vi "Get_reference_samplingdata.vi"(0 "SPU":refnum<k24>, 1 "Ref_monitordata_struct":refnum<k24>[](array[refnum]), 2 "TSL":refnum<k24>, 3 "MPM":refnum<k24>[](array[refnum]), 4 "SOP":i32, 5 "错误输入（无错误）":errorcluster, 6 "STSProcess.PDLSTS":refnum<k24>, 10 "Refdata_struct":refnum<k24>[](array[refnum])) -> (15 "PDLSTS out":refnum<k24>, 19 "error out":errorcluster)   [LabVIEW 2017]
doc: "Get logging reference data & add in"
uses:
  D:/test/PDLSTS/LV_PDL LvVer17.0/LV_PDL_x86/DLL/STSProcess.dll
  DLL/STSProcess.dll
  D:/test/PDLSTS/LV_PDL LvVer17.0/LV_PDL_x86/DLL/InstrumentDLL.dll
  DLL/InstrumentDLL.dll
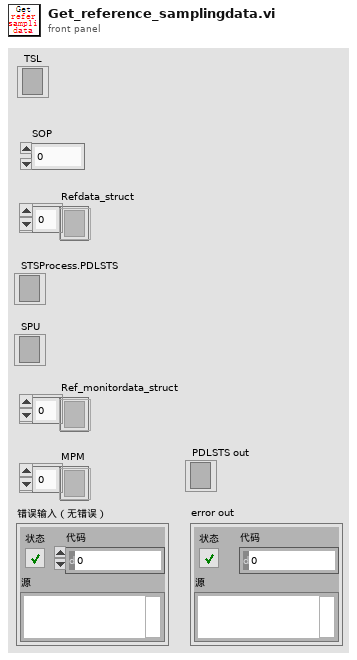
[diagram p1: front panel]
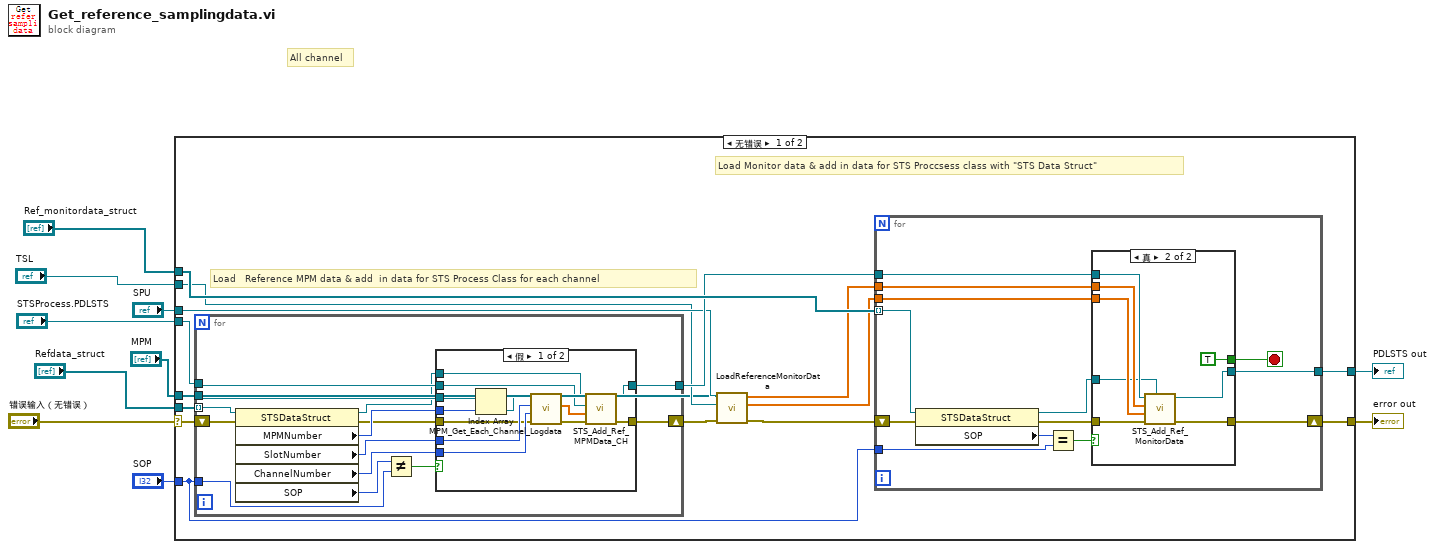
[diagram p0: block diagram]
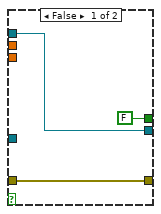
[diagram p2: hidden frame]
diagram:
  # "All channel"
  n1 = case shown="无错误" "错误输入（无错误）" {
    selector: "错误输入（无错误）" -> [w22 w79]
    tunnel: "STSProcess.PDLSTS" -> [w21 w78]
    tunnel: "Ref_monitordata_struct" -> [w25 _]
    tunnel: "SPU" -> [w13 _]
    tunnel: "MPM" -> [w11 _]
    tunnel: "Refdata_struct" -> [w24 _]
    tunnel: [w23 w79] -> w5
    tunnel: [w19 w78] -> w3
    tunnel: "SOP" -> [w18 _]
    tunnel: "TSL" -> [w12 _]
    frame No Error {
      # "Load Monitor data & add in data for STS Proccsess class with \"STS Data Struct\""
      # "Load　Reference MPM data & add  in data for STS Process Class for each channel"
      n2 = for {
        tunnel: w24 -> [w58] mode=indexing
        tunnel: w11 -> [w61]
        tunnel: w21 -> [w59]
        shift-right: [w57] -> w14
        shift-left: w22 -> [w55]
        tunnel: [w53] -> w20
        tunnel: w18 -> [w51]
        n3 = property on="属性节点" class="STSDataStruct"(reference=w58, error in=w55) -> (reference out=w54:refnum<k24>, error out=w56:errorcluster, "MPMNumber"=w60:i32, "SlotNumber"=w63:i32, "ChannelNumber"=w62:i32, "SOP"=w52:i32)
        n4 = Not Equal?(x=w52, y=w51) -> (x != y?=w50:bool)
        n5 = case shown="假" w50 {
          tunnel: w63 -> [w75 _]
          tunnel: w62 -> [w74 _]
          tunnel: w61 -> [w73 _]
          tunnel: w60 -> [w72 _]
          tunnel: w59 -> [w71 w77]
          tunnel: [w70 w76] -> w57
          tunnel: w56 -> [w69 w76]
          tunnel: w54 -> [w65 _]
          tunnel: [w64 w77] -> w53
          frame False {
            n6 = Index Array(array=w73, index=w72) -> (element=w68:refnum<k24>)
            n7 = call "MPM_Get_Each_Channel_Logdata.vi"("error in (no error)"=w69, "channelNumber"=w74, "moduleNumber"=w75, ".NET Reference in"=w68) -> ("error out"=w66:errorcluster, "data out"=w67:sgl[])  [unwired: 5 in, 1 out]
            n8 = call "STS_Add_Ref_MPMData_CH.vi"("错误输入（无错误）"=w66, "data"=w67, "STSProcess.PDSTS"=w71, "Setting"=w65) -> ("错误输出"=w70:errorcluster, "PDLSTS"=w64:refnum<k24>)  [unwired: 6 in]
          }
          frame True {
          }
        }
      }
      n9 = call "LoadReferenceMonitorData.vi"("错误输入（无错误）"=w14, "MPM"=w11, "TSL"=w12, "SPU"=w13) -> ("错误输出"=w15:errorcluster, "monitor"=w16:sgl[], "trigger"=w17:sgl[])  [unwired: 5 in]
      n10 = for {
        tunnel: w25 -> [w33] mode=indexing
        tunnel: w20 -> [w38]
        tunnel: w17 -> [w37]
        tunnel: w16 -> [w36]
        shift-right: [w35] -> w23
        shift-left: w15 -> [w28]
        tunnel: [w34] -> w19
        tunnel: w18 -> [w31]
        stop <- w26 stop-if-true
        n11 = property class="STSDataStruct"(reference=w33, error in=w28) -> (reference out=w29:refnum<k24>, error out=w27:errorcluster, "SOP"=w32:i32)
        n12 = Equal?(x=w32, y=w31) -> (x = y?=w30:bool)
        n13 = case shown="真" w30 {
          tunnel: w38 -> [w41 w49]
          tunnel: w37 -> [_ w48]
          tunnel: w36 -> [_ w47]
          tunnel: w27 -> [w40 w46]
          tunnel: [w40 w45] -> w35
          tunnel: [w41 w44] -> w34
          tunnel: w29 -> [_ w43]
          tunnel: [FALSE TRUE] -> w26
          frame False {
          }
          frame True {
            n14 = call "STS_Add_Ref_MonitorData.vi"("setting"=w43, "错误输入（无错误）"=w46, "monitorData"=w47, "triggerIndex"=w48, "STSProcess.PDLSTS"=w49) -> ("错误输出"=w45:errorcluster, "PDLSTS out"=w44:refnum<k24>)  [unwired: 5 in]
          }
        }
      }
    }
    frame Error {
    }
  }
  "error out" <- w5
  "PDLSTS out" <- w3
